vi "Sub06_MatlabExecuter.vi"(8 "error in (no error)":errorcluster, 11 "Script":string) -> (0 "error out":errorcluster, 2 "matlab standard error":string, 3 "matlab standard output":string)   [LabVIEW 2019]
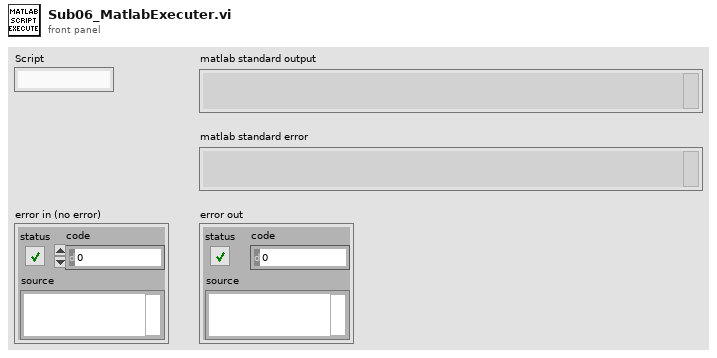
[diagram p1: front panel]
types:
  T1 = enum16{"open", "replace", "create", "open or create", "replace or create", "replace or create with confirmation"}
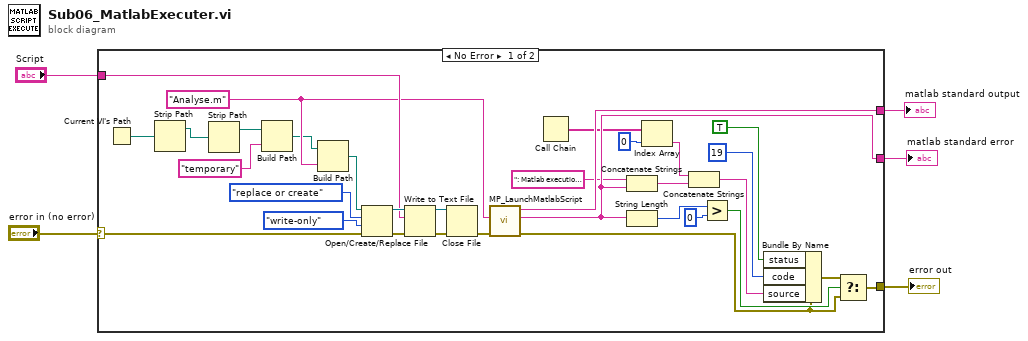
[diagram p0: block diagram]
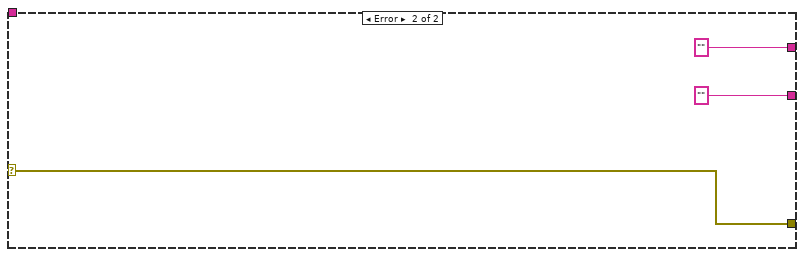
[diagram p2: hidden frame]
diagram:
  n1 = case shown="No Error" "error in (no error)" {
    selector: "error in (no error)" -> [w17 w40]
    tunnel: "Script" -> [w33 _]
    tunnel: [w29 "" ("standard output")] -> w4
    tunnel: [w26 w40] -> w3
    tunnel: [w23 "" ("standard error")] -> w2
    frame No Error {
      w10 = "Analyse.m"
      n2 = Current VI's Path() -> (path=w24:path)
      n3 = Strip Path(path=w24) -> (stripped path=w9:path)  [unwired: 1 out]
      n4 = Strip Path(path=w9) -> (stripped path=w8:path)  [unwired: 1 out]
      n5 = Build Path(base path=w8, name or relative path="temporary") -> (appended path=w6:path)
      n6 = Build Path(base path=w6, name or relative path=w10) -> (appended path=w11:path)
      n7 = Open/Create/Replace File(file path (use dialog)=w11, error in=w17, operation (0:open)=T1."replace or create", access (0:read/write)=enum16{"read/write", "read-only", "write-only"}."write-only") -> (refnum out=w34:refnum<file>, error out=w37:errorcluster)  [unwired: 2 in, 1 out]
      n8 = Write to Text File(file (use dialog)=w34, text=w33, error in=w37) -> (refnum out=w35:refnum<file>, error out=w36:errorcluster)  [unwired: 1 in, 1 out]
      n9 = Close File(refnum=w35, error in=w36) -> (error out=w30:errorcluster)  [unwired: 1 out]
      n10 = call "MP_LaunchMatlabScript.vi"("error in (no error)"=w30, "matlab script name with extension"=w10) -> ("error out"=w19:errorcluster, "standard error"=w23:string, "standard output"=w29:string)  [unwired: 5 in, 2 out]
      n11 = Call Chain() -> (call chain=w14:string[])
      n12 = Concatenate Strings(": Matlab execution error" ("string"), w23) -> (w16:string)
      n13 = String Length(string=w23) -> (length=w21:i32)
      n14 = Index Array(array=w14, index=0) -> (element=w12:string)
      n15 = Concatenate Strings(w12, w16) -> (w15:string)
      n16 = Greater?(x=w21, y=0) -> (0:w27:bool)
      n17 = Bundle By Name(cluster=w19, "status"=TRUE, "code"=19, "source"=w15) -> (w18:errorcluster)
      n18 = Select(t=w18, s=w27, f=w19) -> (s? t:f=w26:errorcluster)
    }
    frame Error {
    }
  }
  "error out" <- w3
  "matlab standard output" <- w4
  "matlab standard error" <- w2
